vi "Graph Set Cursor Mode.vi"(8 "error in":errorcluster, 10 "Cursor Mode":enum32{"Free-Drag", "Single-Plot", "Multi-Plot"}(ring), 11 "Graph Refs in":refnum<vi>[](array[refnum])) -> (0 "error out":errorcluster, 3 "Graph Refs out":refnum<vi>[](array[refnum]))   [LabVIEW 2023, in "FPT_SParam_VST UI.lvlib"]
doc: "Use this VI to update the cursor type on the selected graphs."
uses:
  FPT_SParam_VST UI.lvlib
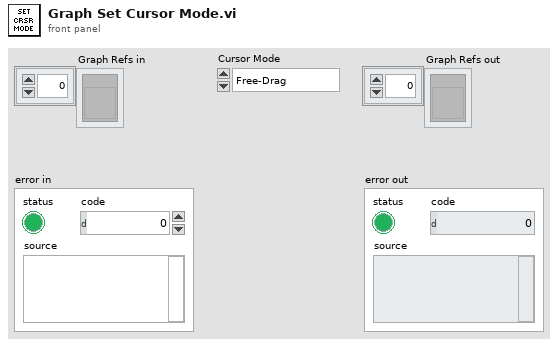
[diagram p1: front panel]
types:
  T1 = typedef "LVCursorListTypeDef.ctl" = cluster{"Name":string, "Color":u32, "Style":u8, "Point Style":u8, "Name Visible":bool, "Allow Drag":bool, "Cursor Mode":u32, "Plot":i32, "Index":i32, "Position":cluster{"X":dbl, "Y":dbl}, "X Scale":u32, "Y Scale":u32, "Watch Plots":i32[], "Watch All Plots":bool, "Plot Area":i32, "Label Offset":cluster{"X":dbl, "Y":dbl}}[]
  T2 = cluster{"Name":string, "Color":u32, "Style":u8, "Point Style":u8, "Name Visible":bool, "Allow Drag":bool, "Cursor Mode":u32, "Plot":i32, "Index":i32, "Position":cluster{"X":dbl, "Y":dbl}, "X Scale":u32, "Y Scale":u32, "Watch Plots":i32[], "Watch All Plots":bool, "Plot Area":i32, "Label Offset":cluster{"X":dbl, "Y":dbl}}
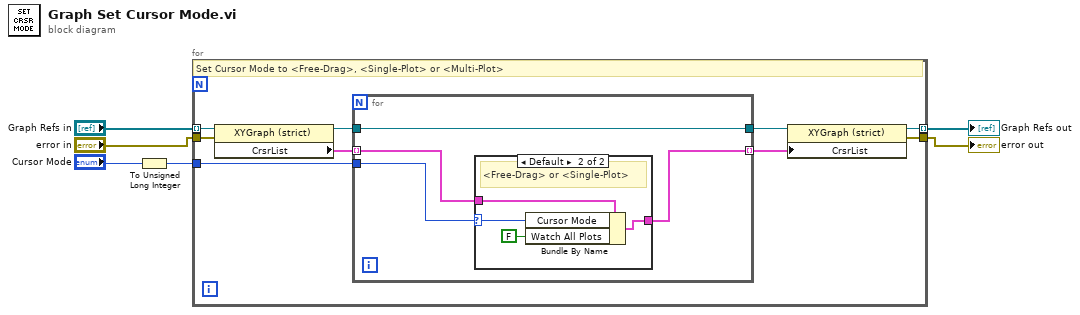
[diagram p0: block diagram]
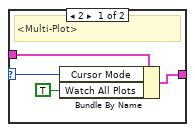
[diagram p2: hidden frame]
diagram:
  n1 = To Unsigned Long Integer(number="Cursor Mode") -> (unsigned 32bit integer=w1:u32)
  n2 = for {
    tunnel: "Graph Refs in" -> [w15] mode=indexing
    tunnel: [w10] -> w3
    tunnel: "error in" -> [w9]
    tunnel: [w8] -> w6 mode=indexing
    tunnel: w1 -> [w7]
    # "Set Cursor Mode to <Free-Drag>, <Single-Plot> or <Multi-Plot>"
    n3 = property class="XYGraph (strict)"(reference=w15, error in=w9) -> (reference out=w14:refnum<vi>, "CrsrList"=w13:T1)  [unwired: 1 out]
    n4 = for {
      tunnel: w14 -> [w17]
      tunnel: w13 -> [w19] mode=indexing
      tunnel: [w18] -> w12 mode=indexing
      tunnel: [w17] -> w11
      tunnel: w7 -> [w16]
      n5 = case shown="Default" w16 {
        selector: w16 -> [w21 w25]
        tunnel: w19 -> [w23 w27]
        tunnel: [w22 w26] -> w18
        frame 2 {
          # "<Multi-Plot>"
          n6 = Bundle By Name(cluster=w23, "Cursor Mode"=w21, "Watch All Plots"=TRUE) -> (w22:T2)
        }
        frame Default {
          # "<Free-Drag> or <Single-Plot>"
          n7 = Bundle By Name(cluster=w27, "Cursor Mode"=w25, "Watch All Plots"=FALSE) -> (w26:T2)
        }
      }
    }
    n8 = property class="XYGraph (strict)"(reference=w11, "CrsrList"=w12) -> (reference out=w8:refnum<vi>, error out=w10:errorcluster)  [unwired: 1 in]
  }
  "Graph Refs out" <- w6
  "error out" <- w3
